vi "test_Write FXP Register Value_Greater Than Maximum.vi"(8 "error in (no error)":errorcluster, 11 "TestCase in":refnum<class "FPGA Register IO Tests.lvclass">=refnum) -> (0 "error out":errorcluster, 3 "TestCase out":refnum<class "FPGA Register IO Tests.lvclass">)   [LabVIEW 2026, in "FPGA Register IO Tests.lvclass"]
uses:
  FPGA Register IO Tests.lvclass
  FPGA Register IO Tests.lvclass/FPGA Register IO Tests.ctl
  APIs/FPGA Register IO/FPGA Register IO.lvlib
  <vilib>/rvi/interface/nirviCloseFPGA/nirviCloseFPGA.xnode
  <vilib>/FPGAPlugInAG/Dynamic/niLvFpga_Close_Dynamic.vi
  <vilib>/fxp/LVFixedPointRepRangeTypeDef.ctl
  <vilib>/fxp/LVFixedPointRepBitsTypeDef.ctl
  APIs/FPGA Register IO/TypeDefs/FXP Configuration.ctl
  <vilib>/Utility/Data Type/NI_Data Type.lvlib
  APIs/FPGA Register IO/Write Methods/Write Data Register/Instances/Write FXP.vi
  Addon/Addon Engine/FPGA Addon Engine.lvlib
  APIs/FPGA Register IO/Read Methods/Read Data Register/Instances/Read FXP.vi
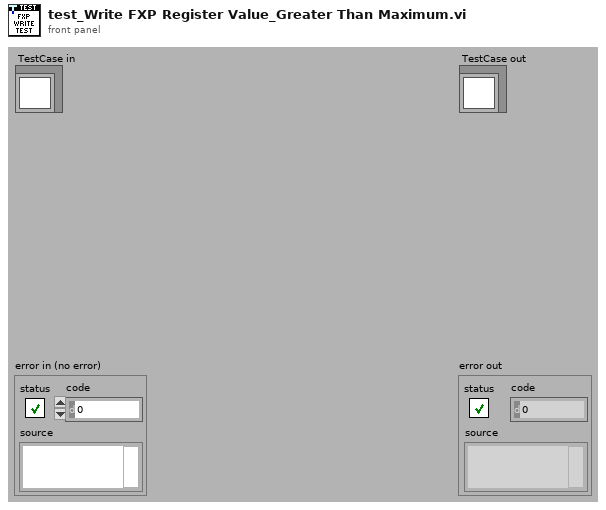
[diagram p1: front panel]
types:
  T1 = typedef "FPGA Register IO.lvlib/FXP Configuration.ctl" = cluster{"FXP Representation":T2, "FXP Range":T3}
  T2 = typedef "LVFixedPointRepBitsTypeDef.ctl" = cluster{"Signed":bool, "Word Length":u32, "Integer Word Length":i32}
  T3 = typedef "LVFixedPointRepRangeTypeDef.ctl" = cluster{"Range Min":dbl, "Range Max":dbl, "Delta":dbl}
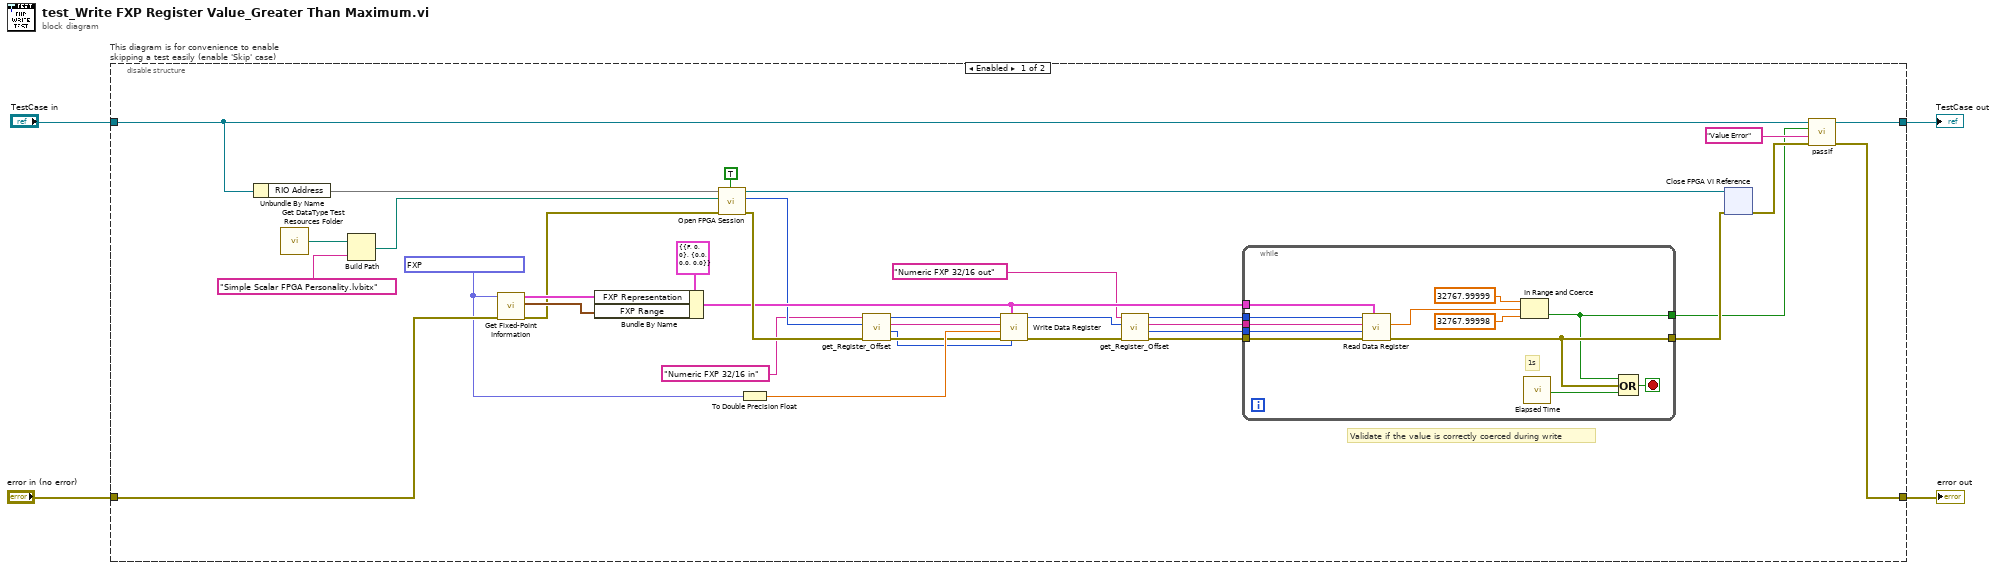
[diagram p0: block diagram]
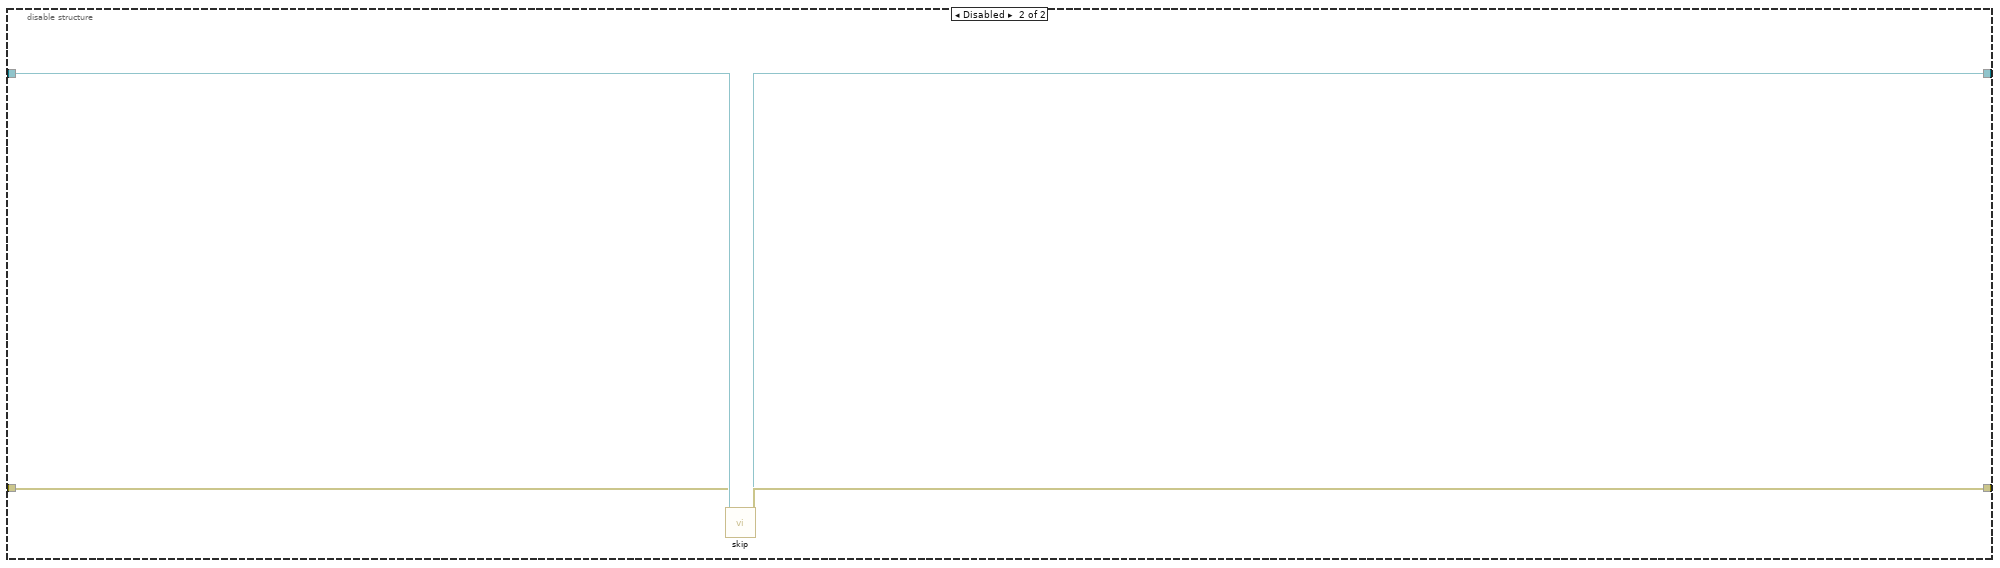
[diagram p2: hidden frame]
diagram:
  n1 = disable-structure "This diagram is for convenience to enable skipping a test easily (enable 'Skip' case)" shown="Enabled" {
    disable-tunnel: "TestCase in" -> [w35 w55]
    disable-tunnel: [w31 w53] -> w1
    disable-tunnel: [w30 w54] -> w3
    disable-tunnel: "error in (no error)" -> [w21 w52]
    frame Enabled {
      w19 = fxp<+/-,32,16> 32767.99998474121 ("value in")
      # "Validate if the value is correctly coerced during write"
      n2 = Unbundle By Name(w35) -> ("RIO Address"=w29)
      n3 = call "Get DataType Test Resources Folder.vi"() -> ("path"=w33:path)
      n4 = Build Path(base path=w33, name or relative path="Simple Scalar FPGA Personality.lvbitx") -> (appended path=w36:path)
      n5 = call <vilib>:"Get Fixed-Point Information.vi"("error in (no error)"=w21, "variant"=w19) -> ("error out"=w20:errorcluster, "FXP range"=w23:T3, "FXP representation"=w24:T2)  [unwired: 6 in, 1 out]
      n6 = Bundle By Name(cluster=T1 {"FXP Representation"={"Signed"=FALSE, "Word Length"=0, "Integer Word Length"=0}, "FXP Range"={"Range Min"=0.0, "Range Max"=0.0, "Delta"=0.0}} ("FXP Configuration"), "FXP Representation"=w24, "FXP Range"=w23) -> (w17:T1)
      n7 = call "Open FPGA Session.vi"("run when loaded (T)"=TRUE ("Run When Loaded (T)"), "error in"=w20, "bitfile path"=w36, "device address"=w29) -> ("error out"=w28:errorcluster, "session out"=w15:u32, "bitfile reference out"=w38:refnum<k20>)  [unwired: 5 in]
      n8 = To Double Precision Float(number=w19) -> (double precision float=w18:dbl)
      n9 = call "get_Register_Offset.vi"("error in (no error)"=w28, "session"=w15, "Name"="Numeric FXP 32/16 in" ("register name")) -> ("error out"=w16:errorcluster, "RegisterOffset"=w11:u32, "Register Name"=w12:string, "session out"=w14:u32)  [unwired: 5 in]
      n10 = call-poly "Write Data Register.vi"("RegisterOffset"=w11, "FXP Configuration"=w17, "error in"=w16, "DBL Value"=w18, "register name"=w12, "session in"=w14) -> ("error out"=w27:errorcluster, "session out"=w9:u32)  [unwired: 4 in]
      n11 = call "get_Register_Offset.vi"("error in (no error)"=w27, "session"=w9, "Name"="Numeric FXP 32/16 out" ("registerName")) -> ("error out"=w10:errorcluster, "RegisterOffset"=w5:u32, "Register Name"=w6:string, "session out"=w8:u32)  [unwired: 5 in]
      n12 = while {
        tunnel: [w48] -> w26
        tunnel: w10 -> [w51]
        tunnel: w8 -> [w50]
        tunnel: w17 -> [w46]
        tunnel: [w42] -> w25
        tunnel: w6 -> [w41]
        tunnel: w5 -> [w40]
        stop <- w49 stop-if-true
        # "1s"
        n13 = call-poly "Read Data Register.vi"("FXP Configuration"=w46, "error in"=w51, "RegisterOffset"=w40, "register name"=w41, "session in"=w50) -> ("error out"=w48:errorcluster, "DBL Value"=w44:dbl)  [unwired: 4 in, 1 out]
        n14 = In Range and Coerce(upper limit=32767.99999 ("y"), x=w44, lower limit=32767.99998 ("y")) -> (In Range?=w42:bool)  [unwired: 1 out]
        n15 = call "Elapsed Time"() -> ("Time has Elapsed"=w47:bool)  [unwired: 12 in, 7 out]
        n16 = Compound Arithmetic op=OR(w42, w48, w47) -> (w49:bool)
      }
      n17 = xnode "Close FPGA VI Reference"("FPGA VI Reference In"=w38, "error in"=w26) -> ("error out"=w34:errorcluster)
      n18 = call-dynamic "passIf.vi"("error in (no error)"=w34, "message (\"\")"="Value Error" ("message (\"\")"), "pass"=w25, "TestCase in"=w35) -> ("error out"=w30:errorcluster, "TestCase out"=w31:refnum<class "FPGA Register IO Tests.lvclass">)  [unwired: 6 in]
    }
    frame Disabled {
      # "skip test result while test is under development"
      n19 = call <vilib>:"skip.vi"("error in (no error)"=w52, "TestCase in"=w55) -> ("error out"=w54:errorcluster, "TestCase out"=w53:refnum<class "FPGA Register IO Tests.lvclass">)  [unwired: 8 in]
    }
  }
  "error out" <- w3
  "TestCase out" <- w1
